vi "Secure-Release Region.vi"(7 "Action":enum16{"Secure", "Release"}(ring), 8 "error in (no error)":errorcluster, 10 "Control In":T1={"I-O.lvclass"=refnum, "Gantry"=refnum, "Dispenser"="COM1"}, 11 "Workspace in":refnum<class "Component Tray.lvclass">) -> (0 "error out":errorcluster, 1 "Position":i32, 2 "Control Out":T1={"I-O.lvclass"=refnum, "Gantry"=refnum, "Dispenser"="COM1"}, 3 "Workspace out":refnum<class "Component Tray.lvclass">)   [LabVIEW 2021, in "Component Tray.lvclass"]
uses:
  Component Tray.lvclass
  C:/Users/HEP/Documents/GitHub/Gantry/UCSB-Gantry-HEP-main/Classes/Workspace/Fixture.lvclass
  Controller/Controllers.ctl
  Controller/I-O/I-O.lvclass
  C:/Program Files (x86)/Aerotech/A3200/LabVIEW/2010/Bin/Aerotech.A3200.dll
  Program Files (x86)/Aerotech/A3200/LabVIEW/2010/Bin/Aerotech.A3200.dll
  Fixture.lvclass/Fixture.ctl
  Read Gantry Region.vi
  Read Position.vi
  Fixture.lvclass
  Component Tray.lvclass/Component Tray.ctl
  Controller/Controller.lvclass
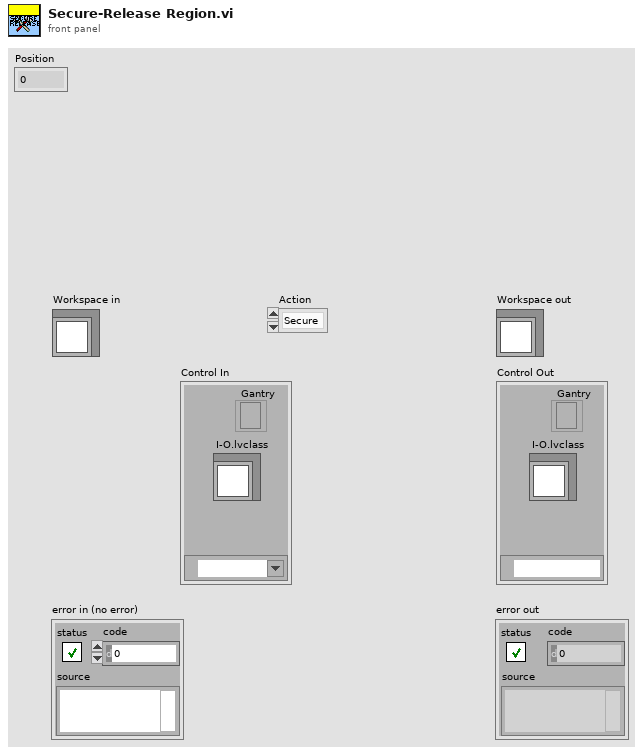
[diagram p1: front panel]
types:
  T1 = typedef "Controller.lvclass/Controllers.ctl" = cluster{"I-O.lvclass":refnum<class "I-O.lvclass">, "Gantry":refnum<k24>, "Dispenser":refnum<visa-resource-name>}
  T2 = typedef "I-O.lvclass/Pin Map.ctl" = cluster{"Region Valves":i32[], "Extra Valves":dbl[][][], "Tool Primary Valve":i32, "Tool Secondary Valve":i32, "Region Sensors":i32[], "Extra Sensors":dbl[][][], "Tool Primary Sensor":dbl, "Tool Secondary Sensor":dbl, "Compression Sensor":dbl, "5V":i32, "Dispenser Sensor":dbl}
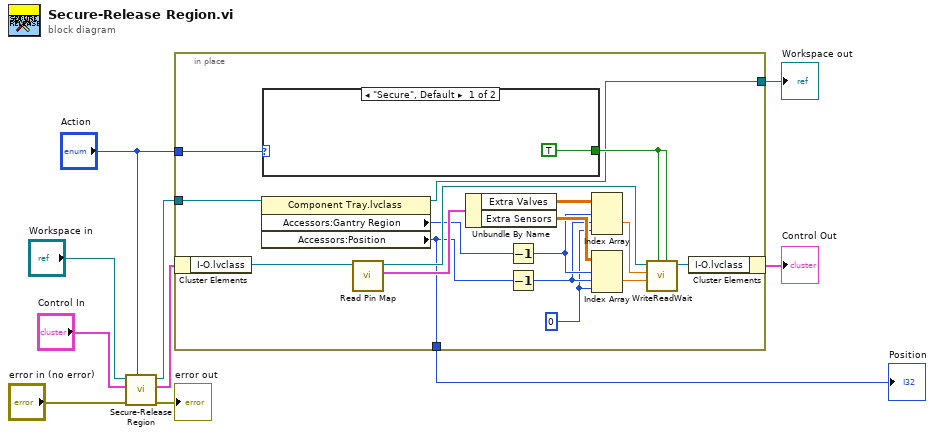
[diagram p0: block diagram]
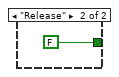
[diagram p2: hidden frame]
diagram:
  n1 = call-parent "Secure-Release Region.vi"("Action"="Action", "error in (no error)"="error in (no error)", "Control In"="Control In", "Fixture in"="Workspace in") -> ("error out"=→"error out":errorcluster, "Control Out"=w6:T1, "Fixture out"=w3:refnum<class "Component Tray.lvclass">)  [unwired: 4 in, 1 out]
  n2 = in-place {
    in-place-border: "Action" -> [w24]
    in-place-border: w3 -> [w21]
    in-place-border: [w15] -> w2
    in-place-border: [w11] -> w1
    w12 = 0
    n3 = in-place-cluster #1(w6) -> ("I-O.lvclass"=w26:refnum<class "I-O.lvclass">)
    n4 = property class="Component Tray.lvclass"(reference=w21) -> (reference out=w15:refnum<class "Component Tray.lvclass">, "Accessors:Gantry Region"=w18:i32, "Accessors:Position"=w11:i32)  [unwired: 1 in, 1 out]
    n5 = case shown="\"Secure\", Default" w24 {
      tunnel: [TRUE FALSE] -> w25
      frame "Secure", Default {
      }
      frame "Release" {
      }
    }
    n6 = call-dynamic "Read Pin Map.vi"("I-O in"=w26) -> ("Pin Map 2"=w27:T2, "I-O out"=w23:refnum<class "I-O.lvclass">)  [unwired: 8 in, 1 out]
    n7 = Unbundle By Name(w27) -> ("Extra Valves"=w20:dbl[][][], "Extra Sensors"=w19:dbl[][][])
    n8 = Decrement(x=w18) -> (x-1=w17:i32)
    n9 = Decrement(x=w11) -> (x-1=w16:i32)
    n10 = Index Array(array=w20, index (dim 0)=w17, index (dim 1)=w16, index (dim 2)=w12) -> (element=w14:dbl)
    n11 = Index Array(array=w19, index (dim 0)=w17, index (dim 1)=w16, index (dim 2)=w12) -> (element=w13:dbl)
    n12 = call "WriteReadWait.vi"("Read Value"=w25, "Write Value"=w25, "Read"=w13, "Write"=w14, "I-O in"=w23) -> ("I-O out"=w22:refnum<class "I-O.lvclass">)  [unwired: 5 in, 1 out]
    n13 = in-place-cluster #1("I-O.lvclass"=w22) -> (→"Control Out":T1)
  }
  "Workspace out" <- w2
  "Position" <- w1
